vi "SCP Open.vi"(8 "Error In":errorcluster, 9 "Password":string, 10 "Username":string, 11 "Hostname or IP":string) -> (0 "Error Out":errorcluster, 2 "Connected?":bool, 3 "SCP Session":refnum<k24>)   [LabVIEW 2020, in "LMH-LINX.lvlib"]
uses:
  LMH-LINX.lvlib
  c:/p4/penguin/lvaddon/MakerHub/LINX/trunk/20.1/objects/MakerHub_LINX/win32U/i386/msvc90/release/LabVIEW/vi.lib/MakerHub/LINX/Resources/Renci.SshNet.dll
  Resources/Renci.SshNet.dll
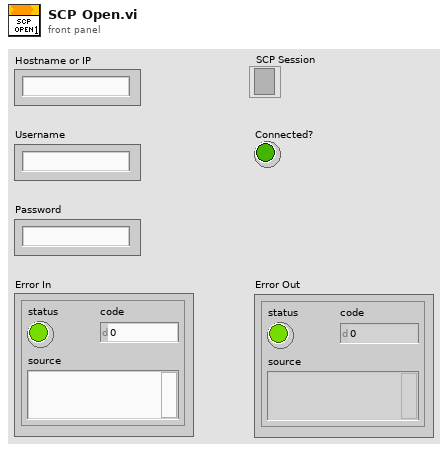
[diagram p1: front panel]
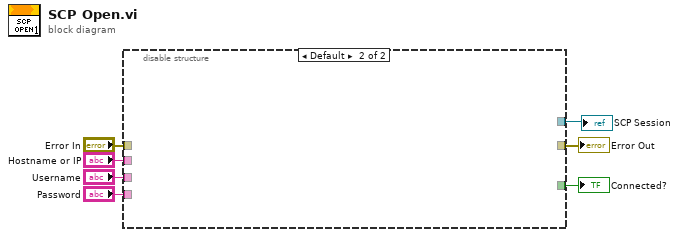
[diagram p0: block diagram]
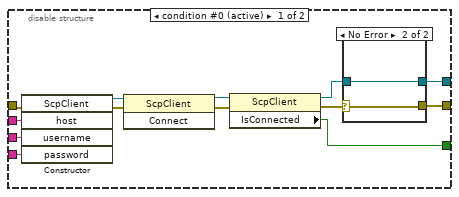
[diagram p2: hidden frame]
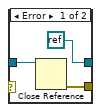
[diagram p3: hidden frame]
diagram:
  n1 = disable-structure shown="Default" {
    disable-tunnel: [w20 _] -> w7
    disable-tunnel: "Error In" -> [w19 _]
    disable-tunnel: "Hostname or IP" -> [w18 _]
    disable-tunnel: "Username" -> [w17 _]
    disable-tunnel: "Password" -> [w16 _]
    disable-tunnel: [w10 _] -> w2
    disable-tunnel: [w8 _] -> w1
    frame condition #0 (active) {
      n2 = constructor class="ScpClient"(error in=w19, "host"=w18, "username"=w17, "password"=w16) -> (reference out=w14:refnum<k24>, error out=w15:errorcluster)  [unwired: 2 in, 4 out]
      n3 = invoke class="ScpClient" method="Connect"(reference=w14, error in=w15) -> (reference out=w13:refnum<k24>, error out=w12:errorcluster)  [unwired: 1 in, 1 out]
      n4 = property class="ScpClient"(reference=w13, error in=w12) -> (reference out=w9:refnum<k24>, error out=w11:errorcluster, "IsConnected"=w20:bool)
      n5 = case shown="No Error" w11 {
        selector: w11 -> [_ w25]
        tunnel: [w22 w25] -> w10
        tunnel: [refnum<k0> refnum w24] -> w8
        tunnel: w9 -> [w21 w24]
        frame Error {
          n6 = Close Reference(reference=w21) -> (error out=w22:errorcluster)  [unwired: 1 in]
        }
        frame No Error {
        }
      }
    }
    frame condition #1 {
    }
  }
  "Error Out" <- w2
  "Connected?" <- w7
  "SCP Session" <- w1
